vi "NISE.Get Property Access.vi"(0 "SLSC Interface in":refnum<class "SLSC Interface.lvclass">, 5 "property":refnum<k21>, 11 "error in (no error)":errorcluster) -> (4 "SLSC Interface out":refnum<class "SLSC Interface.lvclass">, 6 "property out":refnum<k21>, 10 "Prop.Access":i32(ring) items=["None", "Read Only", "Write Only", "Read/Write"], 15 "error out":errorcluster)   [LabVIEW 2016, in "SLSC Interface.lvclass"]
uses:
  SLSC Interface.lvclass
  SLSC Interface.lvclass/SLSC Interface.ctl
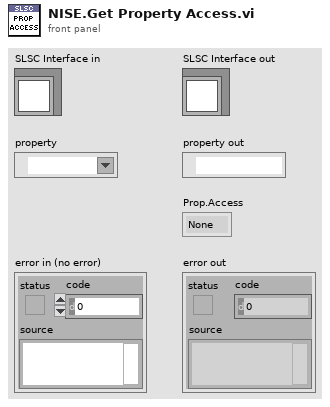
[diagram p1: front panel]
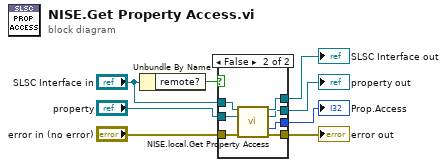
[diagram p0: block diagram]
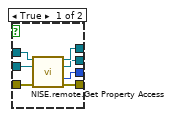
[diagram p2: hidden frame]
diagram:
  n1 = Unbundle By Name("SLSC Interface in") -> ("remote?"=w8:bool)
  n2 = case shown="False" w8 {
    tunnel: "SLSC Interface in" -> [w15 w22]
    tunnel: [w14 w21] -> w7
    tunnel: "property" -> [w13 w20]
    tunnel: [w12 w19] -> w5
    tunnel: [w11 w18] -> w4
    tunnel: "error in (no error)" -> [w10 w17]
    tunnel: [w9 w16] -> w2
    frame True {
      n3 = call "NISE.remote.Get Property Access.vi"("SLSC Remote in"=w15, "property"=w13, "error in (no error)"=w10) -> ("SLSC Remote out"=w14:refnum<class "SLSC Interface.lvclass">, "property out"=w12:refnum<k21>, "Prop.Access"=w11:i32, "error out"=w9:errorcluster)  [unwired: 9 in]
    }
    frame False {
      n4 = call "NISE.local.Get Property Access.vi"("SLSC Local in"=w22, "property"=w20, "error in (no error)"=w17) -> ("SLSC Local out"=w21:refnum<class "SLSC Interface.lvclass">, "property out"=w19:refnum<k21>, "Prop.Access"=w18:i32, "error out"=w16:errorcluster)  [unwired: 9 in]
    }
  }
  "error out" <- w2
  "SLSC Interface out" <- w7
  "property out" <- w5
  "Prop.Access" <- w4
